vi "B-Scan (Timed).vi"(9 "Scan definition":T2={"Max Scan Length"=0, "Update Rate"=1000, "Direction"=enum."Forwards"} {"Update Rate" format="%#_6f"; "Max Scan Length" format="%#_6f"}, 11 "scan data info":T4 {"Error Message" format="%04x"; "Message Header" format="%04x"; "IP"."MIP location" format="%#.0f"; "IP"."Location" format="%#.0f"; "PRF" format="%.0fHz"}) -> (0 "Update Display?":bool, 1 "B-Scan In Progress?":bool, 2 "B-Scan Index":i32, 3 "B-Scan Out":u16[][](array[numeric]))   [LabVIEW 2015]
uses:
  <instrlib>/MicroPulse/Public/Data/Datatypes/MP - scan data info.ctl
  <instrlib>/MicroPulse/Public/Data/Datatypes/MP - data output format.ctl
  <instrlib>/MicroPulse/Public/Data/Datatypes/MP - retain scan.ctl
  <instrlib>/MicroPulse/Public/Data/Datatypes/MP - axis positions (LLC).ctl
  <instrlib>/MicroPulse/Public/Data/Datatypes/MP - fly scan range (timed).ctl
  <instrlib>/MicroPulse/Public/Data/Datatypes/MP - inspection direction.ctl
  <instrlib>/MicroPulse/Public/Helper VIs/Low Level/FGV - B-Scan Active - Action [Enum].ctl
  <instrlib>/MicroPulse/MicroPulse_Driver.lvlib
panel:
  in  "X Scan definition":T1={"Max X Scan Length"=0, "Indexing\nResolution"=1000} {"Indexing\nResolution" format="%#_6f"; "Max X Scan Length" format="%#_6f"}
  # "X-Scan Index"
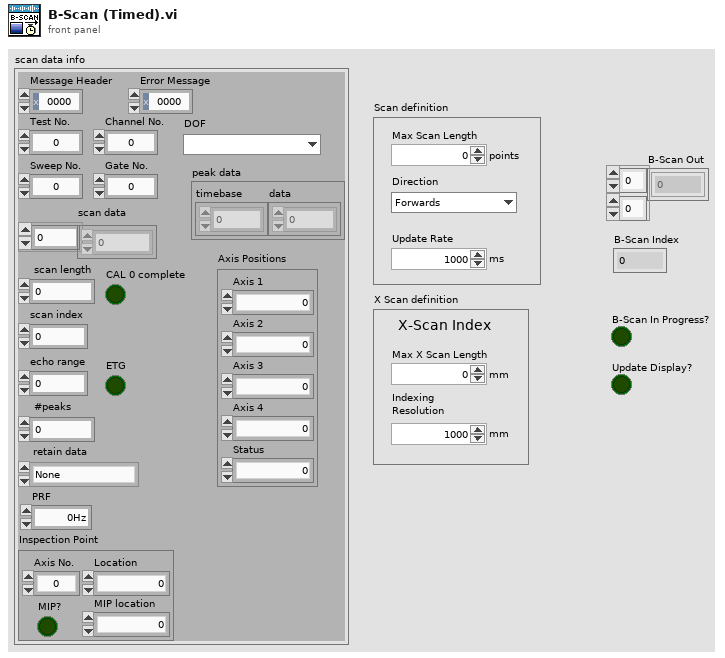
[diagram p1: front panel]
types:
  T1 = cluster{"Max X Scan Length":i32, "Indexing\nResolution":i32}
  T2 = typedef "MicroPulse_Driver.lvlib/MP - fly scan range (timed).ctl" = cluster{"Max Scan Length":i32, "Update Rate":i32, "Direction":T3}
  T3 = typedef "MicroPulse_Driver.lvlib/MP - inspection direction.ctl" = enum16{"Forwards", "Backwards"}
  T4 = typedef "MicroPulse_Driver.lvlib/MP - scan data info.ctl" = cluster{"Message Header":u16, "Error Message":u16, "Test No.":u32, "Channel No.":u8, "Sweep No.":u32, "Gate No.":u32, "DOF":T5, "retain data":T6, "scan data":u16[], "scan length":i32, "scan index":i32, "peak data":cluster{"timebase":u16[], "data":u16[]}, "#peaks":i32, "PRF":dbl, "IP":cluster{"Axis No.":u8, "Location":u32, "MIP location":u32, "MIP?":bool}, "echo range":u16, "ETG":bool, "CAL 0 complete":bool, "Axis Positions":T7}
  T5 = typedef "MicroPulse_Driver.lvlib/MP - data output format.ctl" = enum16{"", "8-bit Mode", "10-bit Mode", "12-bit Mode", "16-bit Mode", "8-bit Log Mode", "12-bit Packed Mode"}
  T6 = typedef "MicroPulse_Driver.lvlib/MP - retain scan.ctl" = enum16{"None", "Ascan", "Peaks"}
  T7 = typedef "MicroPulse_Driver.lvlib/MP - axis positions (LLC).ctl" = cluster{"Axis 1":u32, "Axis 2":u32, "Axis 3":u32, "Axis 4":u32, "Status":u8}
  T8 = typedef "MicroPulse_Driver.lvlib/FGV - B-Scan Active - Action [Enum].ctl" = enum16{"Read", "Read & Reset Start Flag", "Start B-Scan", "B-Scan Finished"}
  T9 = cluster{"Lowest location":i32, "Highest location":i32}
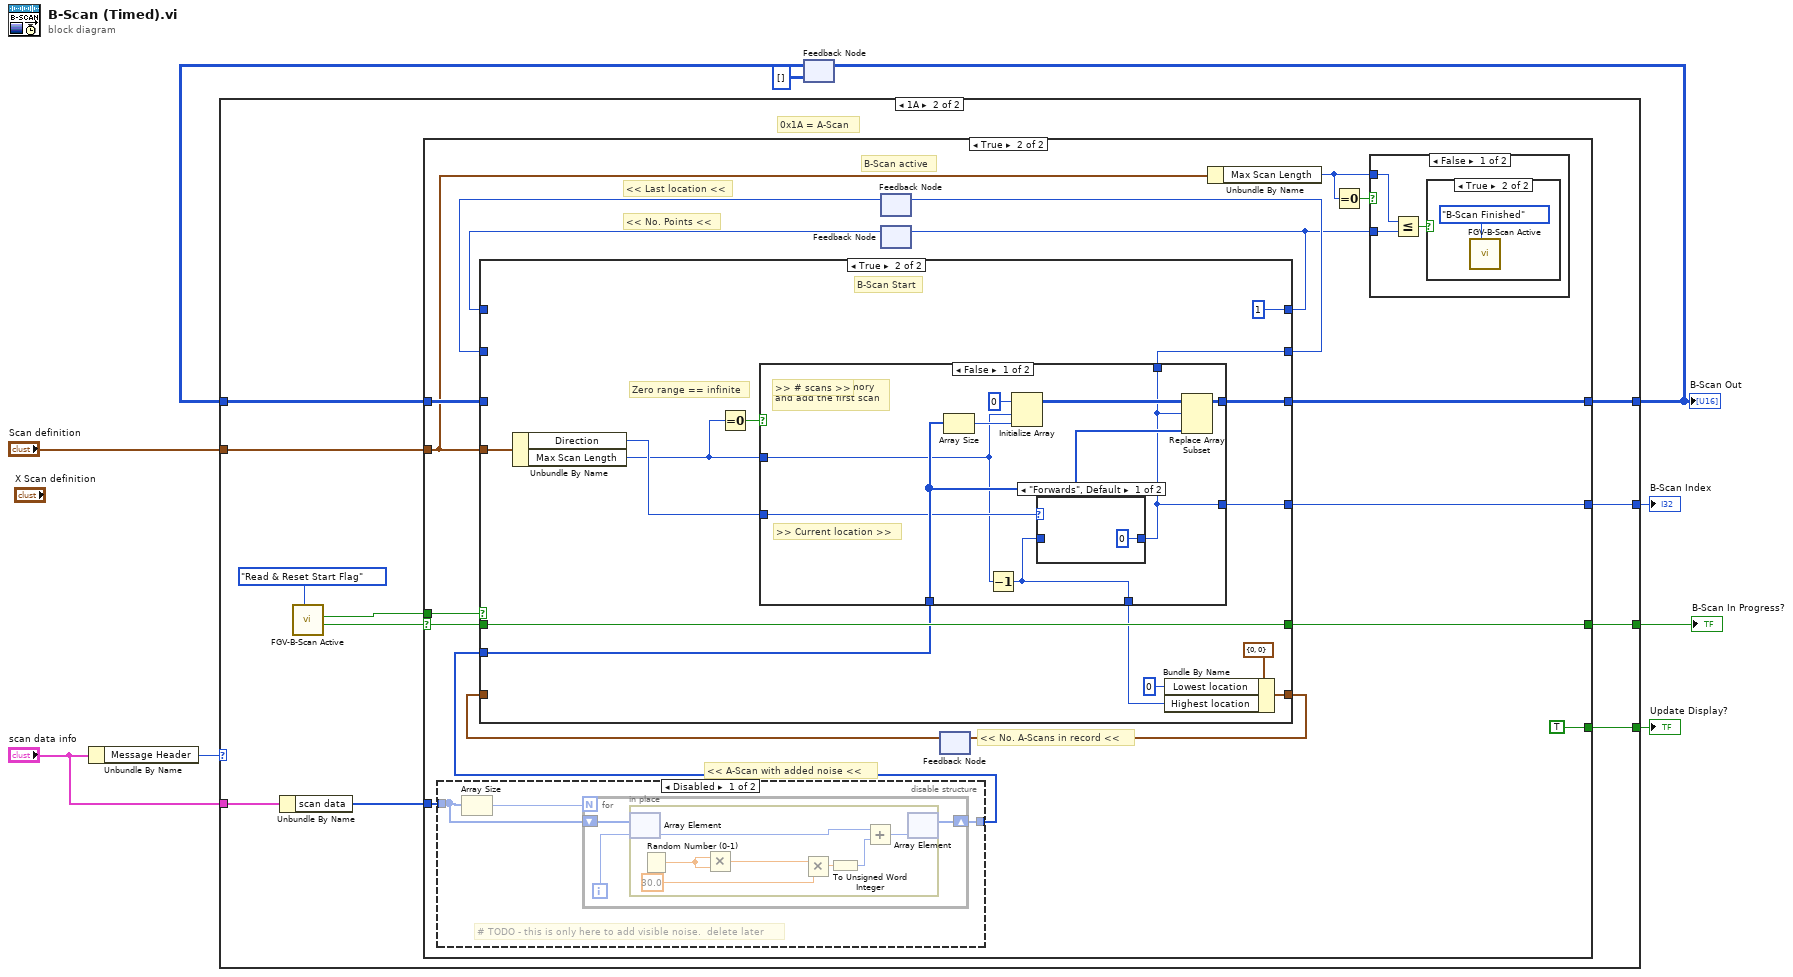
[diagram p0: block diagram]
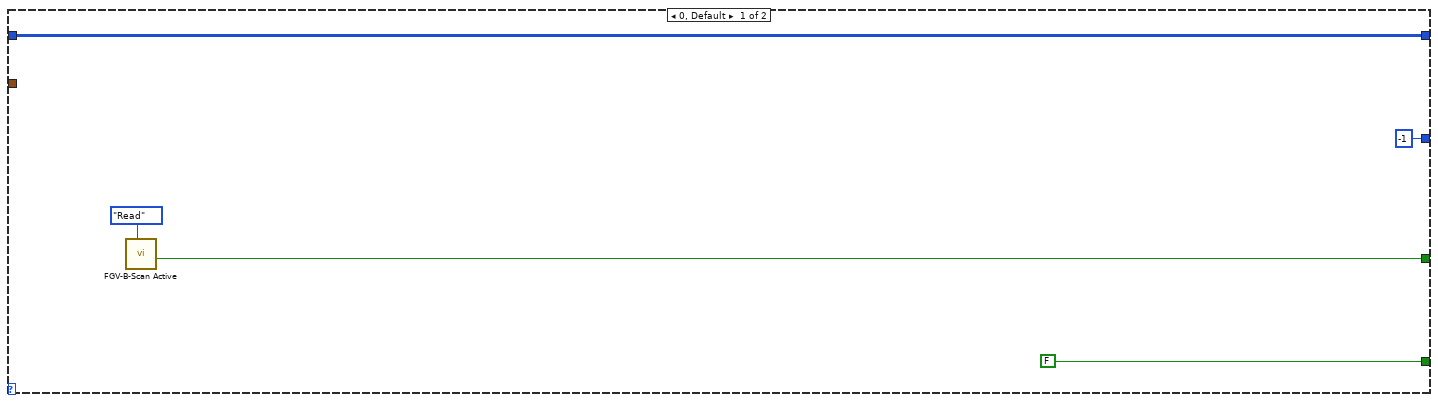
[diagram p2: hidden frame]
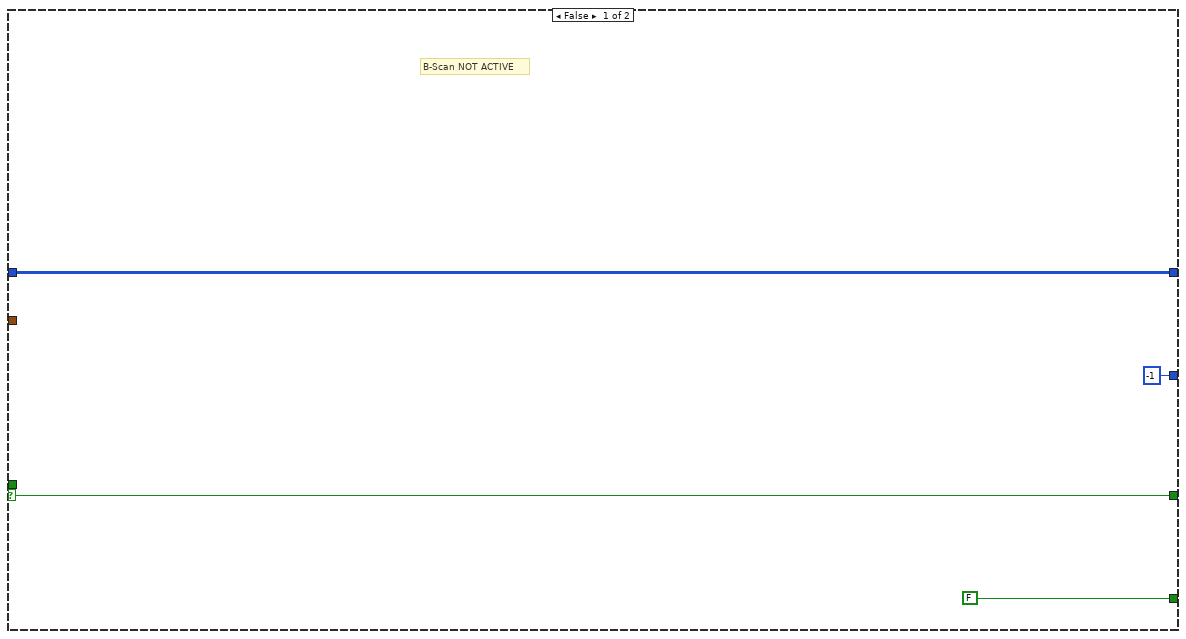
[diagram p3: hidden frame]
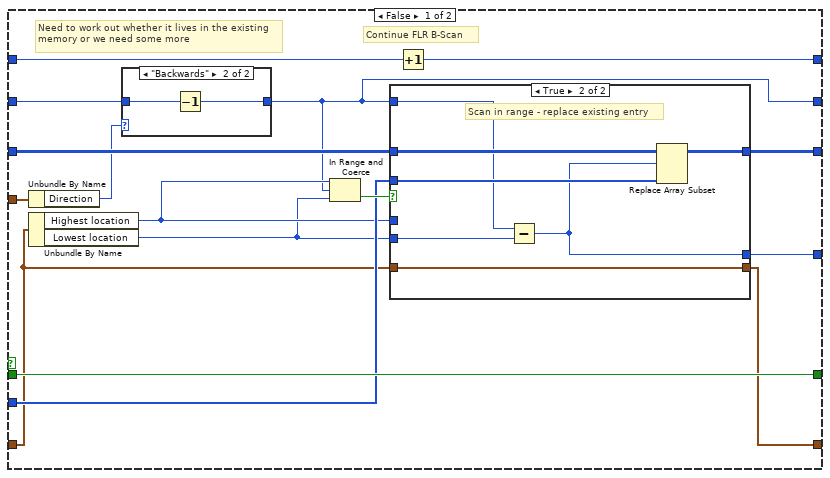
[diagram p7: hidden frame]
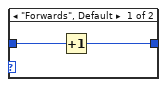
[diagram p8: hidden frame]
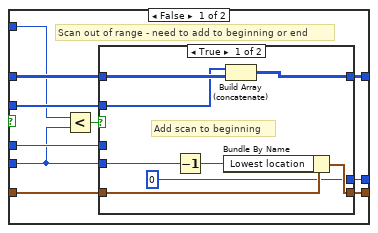
[diagram p9: hidden frame]
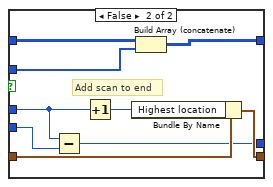
[diagram p10: hidden frame]
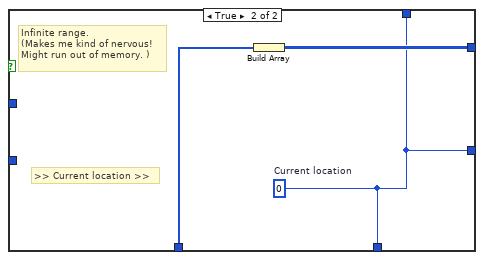
[diagram p12: hidden frame]
diagram:
  n1 = Unbundle By Name("scan data info") -> ("Message Header"=w9:u16)
  n2 = feedback #1(u16[][] []) -> (w6:u16[][])
  n3 = case shown="1A" w9 {
    tunnel: "scan data info" -> [_ w25]
    tunnel: "Scan definition" -> [_ w19]
    tunnel: [w14 w23] -> w7
    tunnel: w6 -> [w14 w22]
    tunnel: [w11 w21] -> w4
    tunnel: [FALSE w20] -> w3
    tunnel: [-1 ("Current location") w15] -> w1
    frame 0, Default {
      n4 = call <instrlib>:"FGV-B-Scan Active.vi"("Action"=FGV_-_B-Scan_Active_-_Action_[Enum]."Read") -> ("B-Scan In Progress?"=w11:bool)  [unwired: 8 in, 2 out]
    }
    frame 26 {
      # "0x1A = A-Scan"
      n5 = Unbundle By Name(w25) -> ("scan data"=w24:u16[])
      n6 = call <instrlib>:"FGV-B-Scan Active.vi"("Action"=FGV_-_B-Scan_Active_-_Action_[Enum]."Read & Reset Start Flag") -> ("B-Scan In Progress?"=w16:bool, "B-Scan Start?"=w17:bool)  [unwired: 8 in, 1 out]
      n7 = case shown="True" w16 {
        selector: w16 -> [w28 w43]
        tunnel: w17 -> [_ w46]
        tunnel: w22 -> [w29 w47]
        tunnel: [w29 w41] -> w23
        tunnel: w24 -> [_ w40]
        tunnel: w19 -> [_ w34]
        tunnel: [w28 w44] -> w21
        tunnel: [FALSE TRUE] -> w20
        tunnel: [-1 ("Current location") w30] -> w15
        frame False {
          # "B-Scan NOT ACTIVE"
        }
        frame True {
          # "<< No. Points <<"
          # "<< Last location <<"
          # "<< A-Scan with added noise <<"
          # "B-Scan active"
          # "<< No. A-Scans in record <<"
          n8 = disable-structure shown="Disabled" {
            disable-tunnel: w40 -> [w49 w61]
            disable-tunnel: [w48 w61] -> w39
            frame Disabled {
              # "# TODO - this is only here to add visible noise.  delete later"
              n9 = Array Size(array=w49) -> (size(s)=w50:i32)
              n10 = for {
                N: w50 -> [_]
                shift-right: [w51] -> w48
                shift-left: w49 -> [w53]
                i -> [w52]
                n11 = in-place {
                  n12 = in-place-array #2(w53, w52) -> (w57:u16)
                  n13 = Random Number (0-1)() -> (number: 0 to 1=w54:dbl)
                  n14 = Multiply(x=w54, y=w54) -> (x*y=w55:dbl)
                  n15 = Multiply(x=w55, y=30.0) -> (x*y=w59:dbl)
                  n16 = To Unsigned Word Integer(number=w59) -> (unsigned 16bit integer=w58:u16)
                  n17 = Add(x=w57, y=w58) -> (x+y=w56:u16)
                  n18 = in-place-array #2(w56) -> (w51:u16[])  [unwired: 1 out]
                }
              }
            }
            frame Enabled {
            }
          }
          n19 = feedback #3() -> (w36:i32)  [unwired: 1 in]
          n20 = feedback #4() -> (w35:i32)  [unwired: 1 in]
          n21 = feedback #5() -> (w45:T9)  [unwired: 1 in]
          n22 = case shown="True" w46 {
            tunnel: w47 -> [w81 _]
            tunnel: [w79 w133] -> w41
            tunnel: w34 -> [w72 w132]
            tunnel: w36 -> [w70 _]
            tunnel: w45 -> [w74 _]
            tunnel: [w80 w131] -> w44
            tunnel: w43 -> [w80 w131]
            tunnel: w39 -> [w77 w130]
            tunnel: [w73 w128] -> w38
            tunnel: [w69 w122] -> w37
            tunnel: [w67 1 ("Current location")] -> w31
            tunnel: w35 -> [w68 _]
            tunnel: [w66 w120] -> w30
            frame False {
              # "Continue FLR B-Scan"
              # "Need to work out whether it lives in the existing memory or we need some more"
              n23 = Unbundle By Name(w72) -> ("Direction"=w71:T3)
              n24 = Unbundle By Name(w74) -> ("Highest location"=w76:i32, "Lowest location"=w75:i32)
              n25 = case shown="\"Backwards\"" w71 {
                tunnel: w70 -> [w83 w85]
                tunnel: [w82 w84] -> w69
                frame "Forwards", Default {
                  n26 = Increment(x=w83) -> (x+1=w82:i32)
                }
                frame "Backwards" {
                  n27 = Decrement(x=w85) -> (x-1=w84:i32)
                }
              }
              n28 = In Range and Coerce(upper limit=w76, x=w69, lower limit=w75) -> (In Range?=w78:bool)  [unwired: 1 out]
              n29 = case shown="True" w78 {
                tunnel: w81 -> [w95 w119]
                tunnel: [w94 w118] -> w79
                tunnel: w69 -> [w92 w116]
                tunnel: w77 -> [w93 w117]
                tunnel: w76 -> [w90 _]
                tunnel: w75 -> [w87 w114]
                tunnel: w74 -> [w89 w115]
                tunnel: [w88 w115] -> w73
                tunnel: [w86 w113] -> w66
                frame False {
                  # "Scan out of range - need to add to beginning or end"
                  n30 = Less?(x=w92, y=w87) -> (x < y?=w91:bool)
                  n31 = case shown="True" w91 {
                    tunnel: w95 -> [w98 w112]
                    tunnel: [w103 w111] -> w94
                    tunnel: w93 -> [w97 w110]
                    tunnel: w90 -> [_ w106]
                    tunnel: w87 -> [w101 w105]
                    tunnel: w89 -> [w102 w109]
                    tunnel: [w99 w107] -> w88
                    tunnel: [0 w104] -> w86
                    frame True {
                      # "Add scan to beginning"
                      n32 = Decrement(x=w101) -> (x-1=w100:i32)
                      n33 = Bundle By Name(cluster=w102, "Lowest location"=w100) -> (w99:T9)
                      n34 = Build Array (concatenate)(w97, w98) -> (w103:u16[][])
                    }
                    frame False {
                      # "Add scan to end"
                      n35 = Subtract(x=w106, y=w105) -> (x-y=w104:i32)
                      n36 = Increment(x=w106) -> (x+1=w108:i32)
                      n37 = Bundle By Name(cluster=w109, "Highest location"=w108) -> (w107:T9)
                      n38 = Build Array (concatenate)(w112, w110) -> (w111:u16[][])
                    }
                  }
                }
                frame True {
                  # "Scan in range - replace existing entry"
                  n39 = Subtract(x=w116, y=w114) -> (x-y=w113:i32)
                  n40 = Replace Array Subset(array=w119, new element=w117, index (row)=w113) -> (w118:u16[][])  [unwired: 1 in]
                }
              }
              n41 = Increment(x=w68) -> (x+1=w67:i32)
            }
            frame True {
              # "Zero range == infinite"
              # "B-Scan Start"
              n42 = Unbundle By Name(w132) -> ("Direction"=w127:T3, "Max Scan Length"=w124:i32)
              n43 = Equal To 0?(x=w124) -> (x = 0?=w125:bool)
              n44 = case shown="False" w125 {
                tunnel: [w139 w147] -> w133
                tunnel: w124 -> [w136 _]
                tunnel: w130 -> [w138 w146]
                tunnel: w127 -> [w137 _]
                tunnel: [w135 w145] -> w126
                tunnel: [w134 w145] -> w122
                tunnel: [w134 w145] -> w120
                frame False {
                  # ">> Current location >>"
                  # "Pre-allocate memory\nand add the first scan"
                  # ">> # scans >>"
                  n45 = Array Size(array=w138) -> (size(s)=w141:i32)
                  n46 = Decrement(x=w136) -> (x-1=w135:i32)
                  n47 = Initialize Array(u16 0 ("index"), w136, w141) -> (w140:u16[][])
                  n48 = case shown="\"Forwards\", Default" w137 {
                    tunnel: w135 -> [_ w144]
                    tunnel: [0 w144] -> w134
                    frame "Forwards", Default {
                    }
                    frame "Backwards" {
                    }
                  }
                  n49 = Replace Array Subset(array=w140, new element=w138, index (row)=w134) -> (w139:u16[][])  [unwired: 1 in]
                }
                frame True {
                  w145 = 0  # Current location
                  # ">> Current location >>"
                  # "Infinite range.\n(Makes me kind of nervous!\nMight run out of memory. )"
                  n50 = Build Array(w146) -> (w147:u16[][])
                }
              }
              n51 = Bundle By Name(cluster=T9 {"Lowest location"=0, "Highest location"=0} ("input cluster"), "Lowest location"=0, "Highest location"=w126) -> (w128:T9)
            }
          }
          n52 = feedback-in #3(w37) -> ()
          n53 = feedback-in #4(w31) -> ()
          n54 = feedback-in #5(w38) -> ()
          n55 = Unbundle By Name(w34) -> ("Max Scan Length"=w32:i32)
          n56 = Equal To 0?(x=w32) -> (x = 0?=w33:bool)
          n57 = case shown="False" w33 {
            tunnel: w32 -> [w63 _]
            tunnel: w31 -> [w64 _]
            frame False {
              n58 = Less Or Equal?(x=w63, y=w64) -> (x <= y?=w62:bool)
              n59 = case shown="True" w62 {
                frame False {
                }
                frame True {
                  n60 = call <instrlib>:"FGV-B-Scan Active.vi"("Action"=FGV_-_B-Scan_Active_-_Action_[Enum]."B-Scan Finished") -> ()  [unwired: 8 in, 3 out]
                }
              }
            }
            frame True {
              # "Do nothing\ninfinite scan"
            }
          }
        }
      }
    }
  }
  "B-Scan Out" <- w7
  "Update Display?" <- w3
  "B-Scan In Progress?" <- w4
  "B-Scan Index" <- w1
  n61 = feedback-in #1(w7) -> ()
